vi "ROI grp-Check if all ROIs group are visible.vi"(8 "error in (no error)":errorcluster) -> (0 "error out":errorcluster, 2 "Group's ROIs are all visible":bool)   [LabVIEW 2017]
uses:
  Global variables/gl_Functional Imaging-Global variables.vi
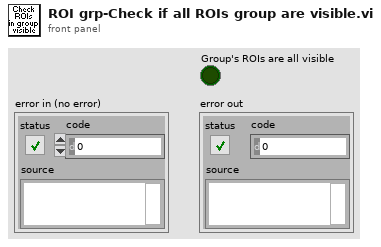
[diagram p1: front panel]
types:
  T1 = typedef "Functional Imging UI Refs.ctl" = cluster{"Menu ref":refnum<k9>, "Image control":refnum<vi>, "VI ref":refnum<vi>, "XGrapher":refnum<vi>, "Smoothing":refnum<vi>, "POI Averaging":refnum<vi>, "Normalize":refnum<vi>, "POI data points in each trial":refnum<vi>, "Channel":refnum<vi>, "Experiment data folder path":refnum<vi>, "[ROI vis]":refnum<vi>, "[Groups] visbl":T2, "Group Name":refnum<vi>, "POI index":refnum<vi>, "Trial No.":refnum<vi>, "Intensity Zoom":refnum<vi>, "Trial Cursor Enabled":refnum<vi>, "Number of Trials (ind 1)":refnum<vi>, "Number of Trials (ind 2)":refnum<vi>, "MiniScans Available":refnum<vi>, "POI Available":refnum<vi>, "Defer graph updates":refnum<vi>, "Waveform selector":refnum<vi>, "#of selected POI":refnum<vi>, "#of selected MiniScans":refnum<vi>, "#of selected groups":refnum<vi>, "Max Z-Projection":refnum<vi>, "Z-Plane Selector":refnum<vi>, "Index of miniscan point to visualise":refnum<vi>, "ROI vis. mode":refnum<vi>, "Total # of points":refnum<vi>, "Index of group clicked on":refnum<vi>, "Pane 1":refnum<vi>, "Pane 2":refnum<vi>, "Pane 3":refnum<vi>, "Pane 4":refnum<vi>, "Pane 5":refnum<vi>, "Pane 6":refnum<vi>, "Deselect all ROI":refnum<vi>, "Deselect all groups":refnum<vi>}
  T2 = typedef "Groups array referecne.ctl" = refnum<vi>
  T3 = typedef "ROI selector array-ROI vis.ctl" = T4[]
  T4 = typedef "Interface-ROI selection cluster.ctl" = cluster{"ROI number":i32, "ROI ID":T5, "Visibility":bool}
  T5 = typedef "ROI ID Enum.ctl" = enum16{"Point", "MiniScan", "Comp. MiniScan", "Rectangle", "Comp. volume", "Arb. plane point"}
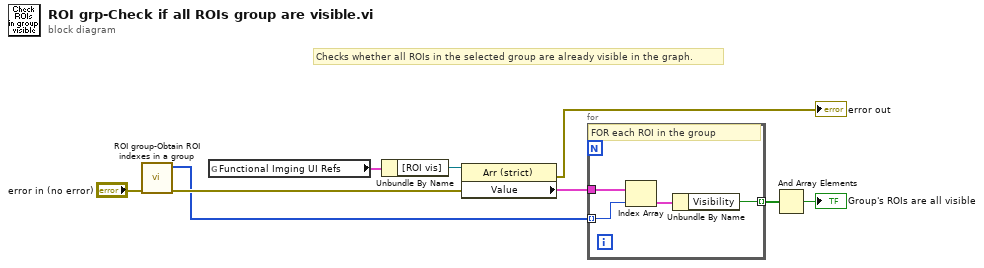
[diagram p0: block diagram]
diagram:
  # "Checks whether all ROIs in the selected group are already visible in the graph."
  n1 = call "ROI group-Obtain ROI indexes in a group.vi"("error in (no error)"="error in (no error)") -> ("error out"=w5:errorcluster, "Group's ROIs indexes"=w4:i32[])  [unwired: 9 in]
  n2 = global read "gl_Functional Imaging-Global variables.vi" "Functional Imging UI Refs"() -> (w6:T1)
  n3 = Unbundle By Name(w6) -> ("[ROI vis]"=w7:refnum<vi>)
  n4 = property on="Property Node" class="Arr (strict)"(reference=w7, error in=w5) -> (error out=→"error out":errorcluster, "Value"=w3:T3)  [unwired: 1 out]
  n5 = for {
    tunnel: w4 -> [w13] mode=indexing
    tunnel: w3 -> [w12]
    tunnel: [w10] -> w2 mode=indexing
    # "FOR each ROI in the group"
    n6 = Index Array(array=w12, index=w13) -> (element=w11:T4)
    n7 = Unbundle By Name(w11) -> ("Visibility"=w10:bool)
  }
  n8 = And Array Elements(Boolean array=w2) -> (logical AND=→"Group's ROIs are all visible":bool)
